vi "SPARK Frames FGV.vi"(7 "Action":T7(ring), 10 "Periodic Status":T1, 11 "MotorControlDeviceRef":T2={"DeviceStatus"={"status"=FALSE, "code"=0, "source"=""}, "Type"=enum."PWM", "PWM"={"PWM Channel"=enum."Invalid", "DeadBand"={"Name"="", "maxPositivePwm"=0, "minPositivePwm"=0, "centerPwm"=0, "maxNegativePwm"=0, "minNegativePwm"=0, "angularRange"=0}}, "CAN"={"Device Number"=0, "SetOutput VI Ref"=variant, "GetOutput VI Ref"=variant, "Enable VI Ref"=variant, "Disable VI Ref"=variant, "Data"=variant}, "Invert"=FALSE, "DIO PWM"={"PWM \"Enable\" Channel"=enum."Invalid", "DIOChannel"=enum."Invalid", "PWM Rate"=0.0}}) -> (3 "Map":map{T2, u16}(c390))   [LabVIEW 2023]
uses:
  <vilib>/Rock Robotics/WPI/MotorControl/WPI_MotorControlDeviceRef.ctl
  <vilib>/Rock Robotics/WPI/MotorControl/WPI_MotorControlType.ctl
  <vilib>/Rock Robotics/SystemInterfaces/DIO/FPGA_DIOPWMChannel.ctl
  <vilib>/Rock Robotics/WPI/PWM/WPI_PWMDeadband.ctl
  <vilib>/Rock Robotics/SystemInterfaces/DIO/FPGA_DIOChannel.ctl
  Typedef/SPARK Periodic Status.ctl
  <vilib>/Utility/miscctls.llb/LVMapReplaceAction.ctl
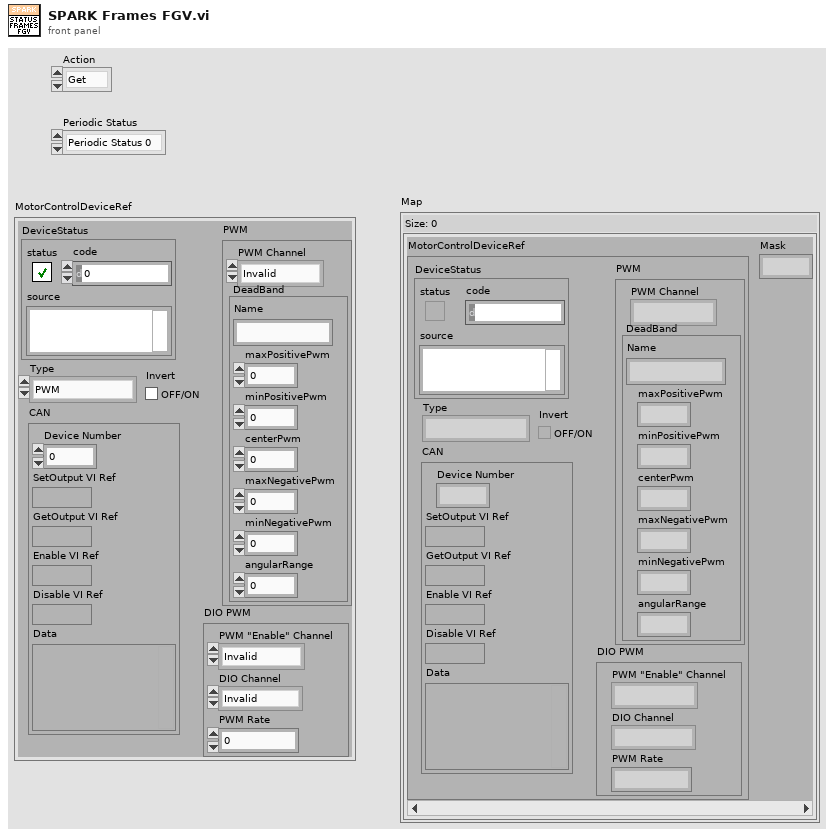
[diagram p1: front panel]
types:
  T1 = typedef "SPARK Periodic Status.ctl" = enum16{"Periodic Status 0", "Periodic Status 1", "Periodic Status 2", "Periodic Status 3", "Periodic Status 4", "Periodic Status 5", "Periodic Status 6", "Periodic Status 7", "Periodic Status 8", "Periodic Status 9"}
  T2 = typedef "WPI_MotorControlDeviceRef.ctl" = cluster{"DeviceStatus":errorcluster, "Type":T3, "PWM":cluster{"PWM Channel":T4, "DeadBand":T5}, "CAN":cluster{"Device Number":u8, "SetOutput VI Ref":variant, "GetOutput VI Ref":variant, "Enable VI Ref":variant, "Disable VI Ref":variant, "Data":variant}, "Invert":bool, "DIO PWM":cluster{"PWM \"Enable\" Channel":T4, "DIOChannel":T6, "PWM Rate":dbl}}
  T3 = typedef "WPI_MotorControlType.ctl" = enum16{"PWM", "CAN", "DIO PWM"}
  T4 = typedef "FPGA_DIOPWMChannel.ctl" = enum8{"PWM 0", "PWM 1", "PWM 2", "PWM 3", "PWM 4", "PWM 5", "PWM 6", "PWM 7", "PWM 8", "PWM 9", "PWM MXP 0", "PWM MXP 1", "PWM MXP 2", "PWM MXP 3", "PWM MXP 4", "PWM MXP 5", "PWM MXP 6", "PWM MXP 7", "PWM MXP 8", "PWM MXP 9", "Invalid"}
  T5 = typedef "WPI_PWMDeadband.ctl" = cluster{"Name":string, "maxPositivePwm":i32, "minPositivePwm":i32, "centerPwm":i32, "maxNegativePwm":i32, "minNegativePwm":i32, "angularRange":u16}
  T6 = typedef "FPGA_DIOChannel.ctl" = enum8{"DIO 0", "DIO 1", "DIO 2", "DIO 3", "DIO 4", "DIO 5", "DIO 6", "DIO 7", "DIO 8", "DIO 9", "DIO MXP 0", "DIO MXP 1", "DIO MXP 2", "DIO MXP 3", "DIO MXP 4", "DIO MXP 5", "DIO MXP 6", "DIO MXP 7", "DIO MXP 8", "DIO MXP 9", "DIO MXP 10", "DIO MXP 11", "DIO MXP 12", "DIO MXP 13", "DIO MXP 14", "DIO MXP 15", "SPI Port CS1", "SPI Port CS2", "SPI Port CS3", "SPI Port MISO", "SPI Port MOSI", "Invalid"}
  T7 = enum16{"Get", "Add frame", "Remove frame", "Clear all frames", "Clear device"}
  T8 = typedef "LVMapReplaceAction.ctl" = enum32{"Modify Entry only if found", "Add or Modify Entry", "Delete Entry"}
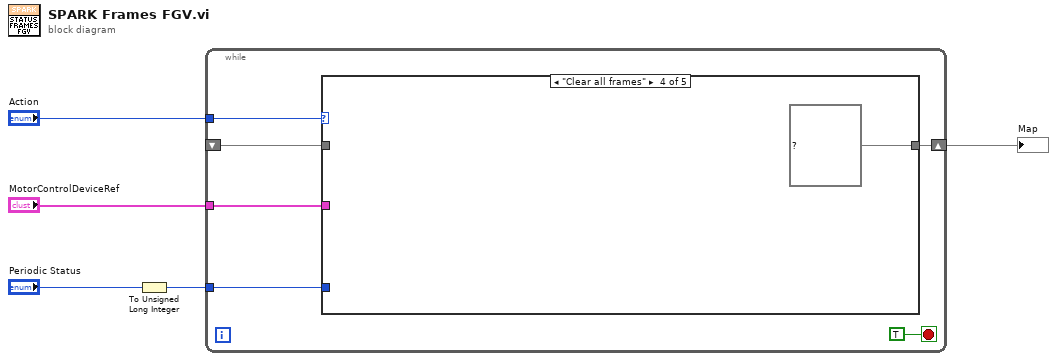
[diagram p0: block diagram]
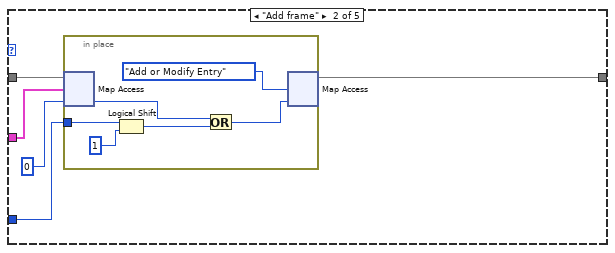
[diagram p3: hidden frame]
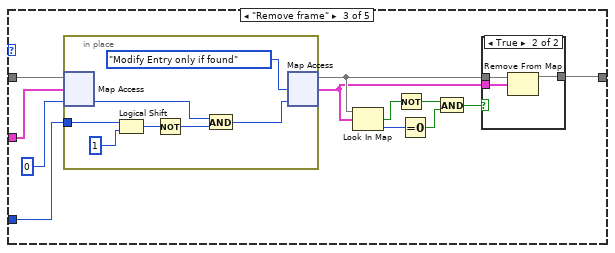
[diagram p4: hidden frame]
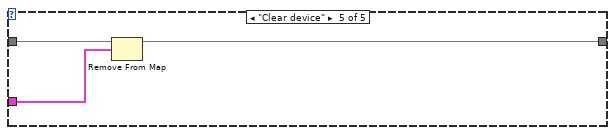
[diagram p6: hidden frame]
diagram:
  n1 = To Unsigned Long Integer(number="Periodic Status") -> (unsigned 32bit integer=w2:u32)
  n2 = while {
    shift-right: [w9] -> w1
    shift-left: _ -> [w8]
    tunnel: "Action" -> [w10]
    tunnel: w2 -> [w7]
    tunnel: "MotorControlDeviceRef" -> [w6]
    stop <- TRUE stop-if-true
    n3 = case shown="\"Clear all frames\"" w10 {
      tunnel: [w12 w13 w24 map{T2, u16} {} ("Map") w48] -> w9
      tunnel: w8 -> [w12 w16 w34 _ w50]
      tunnel: w7 -> [_ w15 w33 _ _]
      tunnel: w6 -> [_ w17 w35 _ w49]
      frame "Get" {
      }
      frame "Add frame" {
        n4 = in-place {
          in-place-border: w15 -> [w20]
          n5 = in-place-map #1(w16, w17, u32 0) -> (w21:u16)  [unwired: 1 out]
          n6 = Logical Shift(y=w20, x=u32 1) -> (x << y=w19:u32)
          n7 = Or(x=w21, y=w19) -> (x .or. y?=w23:u32)
          n8 = in-place-map #1(w23, LVMapReplaceAction."Add or Modify Entry" ("action")) -> (w13:map{T2, u16})  [unwired: 2 out]
        }
      }
      frame "Remove frame" {
        n9 = in-place {
          in-place-border: w33 -> [w43]
          n10 = in-place-map #2(w34, w35, u32 0) -> (w44:u16)  [unwired: 1 out]
          n11 = Logical Shift(y=w43, x=u32 1) -> (x << y=w42:u32)
          n12 = Not(x=w42) -> (.not. x?=w40:u32)
          n13 = And(x=w44, y=w40) -> (x .and. y?=w46:u32)
          n14 = in-place-map #2(w46, LVMapReplaceAction."Modify Entry only if found" ("action")) -> (w27:map{T2, u16}, w26:T2)  [unwired: 1 out]
        }
        n15 = Look In Map(map=w27, key=w26) -> (key not found?=w31:bool, value=w29:u16)  [unwired: 1 in]
        n16 = Not(x=w31) -> (.not. x?=w30:bool)
        n17 = Equal To 0?(x=w29) -> (x = 0?=w28:bool)
        n18 = And(x=w30, y=w28) -> (x .and. y?=w25:bool)
        n19 = case shown="True" w25 {
          tunnel: w27 -> [w36 w39]
          tunnel: w26 -> [_ w38]
          tunnel: [w36 w37] -> w24
          frame False {
          }
          frame True {
            n20 = Remove From Map(10:w38, 11:w39) -> (3:w37:map{T2, u16})  [unwired: 2 out]
          }
        }
      }
      frame "Clear all frames" {
      }
      frame "Clear device" {
        n21 = Remove From Map(10:w49, 11:w50) -> (3:w48:map{T2, u16})  [unwired: 2 out]
      }
    }
  }
  "Map" <- w1
